vi "Agilent N6700 Series Configure Voltage.vi"() -> ()   [LabVIEW 2016]
doc: "Configures the power supply's output range on a channel, configures the DC voltage level, channel appears at the output connector and takes a measurement on the output signal and returns the measured value."
uses:
  <instrlib>/Agilent N6700 Series/Agilent N6700 Series.lvlib
panel:
  in  "Limit (1.0 A)":dbl=1.0 format="%^.3e"
  in  "Behavior (0: Regulatory Limit)":i32(ring) items=["Regulatory Limit", "Trip Limit"]
  out "Voltage Measurement":dbl format="%^.3e"
  in  "Voltage Level  (5.0 V)":dbl=5.0 format="%^.3e"
  in  "Voltage Range (10.0 V)":dbl=10.0 format="%^.3e"
  in  "Channel Name (1)":string="1"
  in  "VISA resource name":refnum<visa-resource-name>
  # "(c) 2004-2019  National Instruments.  ALL RIGHTS RESERVED."
  # "Agilent N6700 DC Power Supply"
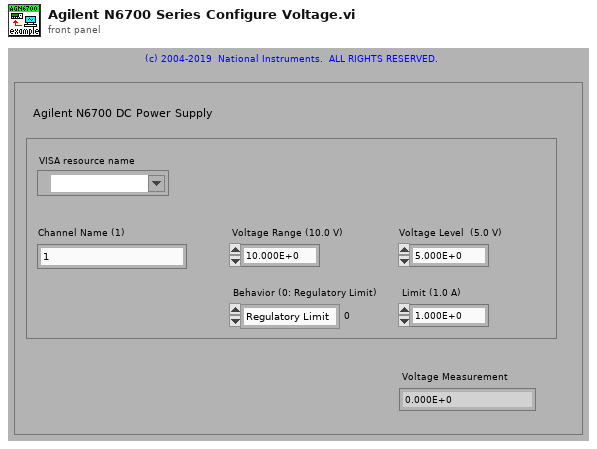
[diagram p1: front panel]
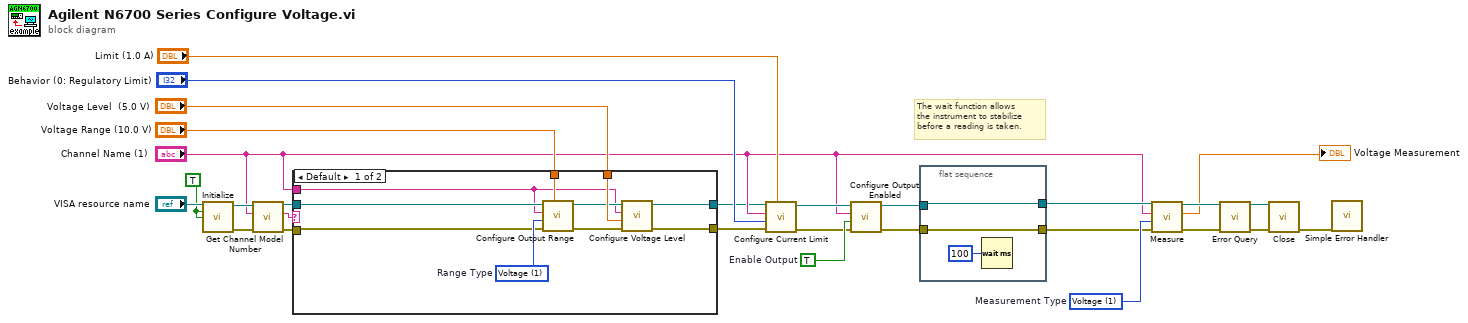
[diagram p0: block diagram]
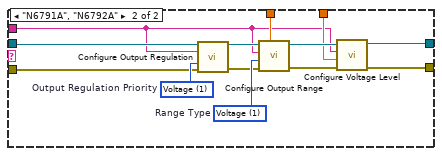
[diagram p2: hidden frame]
diagram:
  w18 = TRUE ("Reset? (T: Yes)")
  w19 = 1 items=["Voltage"=1, "Current"=0]  # Measurement Type
  w20 = TRUE  # Enable Output
  # "The wait function allows \nthe instrument to stabilize\nbefore a reading is taken."
  n1 = call <instrlib>:"Initialize.vi"("VISA resource name"="VISA resource name", "ID Query? (T: Yes)"=w18, "Reset? (T: Yes)"=w18) -> ("VISA resource name out"=w9:refnum<visa-resource-name>, "error out"=w8:errorcluster)  [unwired: 11 in]
  n2 = call <instrlib>:"Get Channel Model Number.vi"("error in (no error)"=w8, "Channel Name (1)"="Channel Name (1)", "VISA resource name"=w9) -> ("error out"=w6:errorcluster, "Model Number"=w5:string, "VISA resource name out"=w7:refnum<visa-resource-name>)  [unwired: 6 in]
  n3 = case shown="Default" w5 {
    tunnel: "Voltage Range (10.0 V)" -> [w35 w51]
    tunnel: "Channel Name (1)" -> [w29 w41]
    tunnel: w7 -> [w37 w46]
    tunnel: w6 -> [w36 w45]
    tunnel: "Voltage Level  (5.0 V)" -> [w33 w42]
    tunnel: [w31 w39] -> w2
    tunnel: [w30 w40] -> w1
    frame Default {
      w38 = 1 items=["Voltage"=1, "Current"=0]  # Range Type
      n4 = call <instrlib>:"Configure Output Range.vi"("Range (0.0)"=w35, "error in (no error)"=w36, "Range Type (1: Voltage)"=w38, "Channel Name (1)"=w29, "VISA resource name"=w37) -> ("error out"=w34:errorcluster, "VISA resource name out"=w32:refnum<visa-resource-name>)  [unwired: 5 in]
      n5 = call <instrlib>:"Configure Voltage Level.vi"("error in (no error)"=w34, "Level  (0.0 volts)"=w33, "Channel Name (1)"=w29, "VISA resource name"=w32) -> ("error out"=w31:errorcluster, "VISA resource name out"=w30:refnum<visa-resource-name>)  [unwired: 6 in]
    }
    frame "N6791A", "N6792A" {
      w47 = 1 items=["Voltage"=1, "Current"=0]  # Output Regulation Priority
      w50 = 1 items=["Voltage"=1, "Current"=0]  # Range Type
      n6 = call <instrlib>:"Configure Output Regulation.vi"("VISA resource name"=w46, "Channel Name (1)"=w41, "Output Regulation Priority (1: Voltage)"=w47, "error in (no error)"=w45) -> ("VISA resource name out"=w49:refnum<visa-resource-name>, "error out"=w48:errorcluster)  [unwired: 10 in]
      n7 = call <instrlib>:"Configure Output Range.vi"("Range (0.0)"=w51, "error in (no error)"=w48, "Range Type (1: Voltage)"=w50, "Channel Name (1)"=w41, "VISA resource name"=w49) -> ("error out"=w43:errorcluster, "VISA resource name out"=w44:refnum<visa-resource-name>)  [unwired: 5 in]
      n8 = call <instrlib>:"Configure Voltage Level.vi"("error in (no error)"=w43, "Level  (0.0 volts)"=w42, "Channel Name (1)"=w41, "VISA resource name"=w44) -> ("error out"=w39:errorcluster, "VISA resource name out"=w40:refnum<visa-resource-name>)  [unwired: 6 in]
    }
  }
  n9 = call <instrlib>:"Configure Current Limit.vi"("Limit (0.0 amps)"="Limit (1.0 A)", "error in (no error)"=w2, "Behavior (0: Regulatory Limit)"="Behavior (0: Regulatory Limit)", "Channel Name (1)"="Channel Name (1)", "VISA resource name"=w1) -> ("error out"=w17:errorcluster, "VISA resource name out"=w16:refnum<visa-resource-name>)  [unwired: 5 in]
  n10 = call <instrlib>:"Configure Output Enabled.vi"("error in (no error)"=w17, "Enable Output (False)"=w20, "Channel Name (1)"="Channel Name (1)", "VISA resource name"=w16) -> ("error out"=w10:errorcluster, "VISA resource name out"=w13:refnum<visa-resource-name>)  [unwired: 6 in]
  n11 = flat-sequence {
    tunnel: w13 -> [w54]
    tunnel: [w54] -> w12
    tunnel: [w52] -> w11
    tunnel: w10 -> [w52]
    frame #0 {
      n12 = Wait (ms)(milliseconds to wait=u32 100) -> ()  [unwired: 1 out]
    }
  }
  n13 = call <instrlib>:"Measure.vi"("error in (no error)"=w11, "Measurement Type (1: Voltage)"=w19, "Channel Name (1)"="Channel Name (1)", "VISA resource name"=w12) -> ("error out"=w27:errorcluster, "Measurement"=→"Voltage Measurement":dbl, "VISA resource name out"=w24:refnum<visa-resource-name>)  [unwired: 5 in]
  n14 = call <instrlib>:"Error Query.vi"("VISA resource name"=w24, "error in (no error)"=w27) -> ("VISA resource name out"=w25:refnum<visa-resource-name>, "error out"=w26:errorcluster)  [unwired: 10 in, 2 out]
  n15 = call <instrlib>:"Close.vi"("VISA resource name"=w25, "error in (no error)"=w26) -> ("error out"=w28:errorcluster)  [unwired: 13 in]
  n16 = call <vilib>:"Simple Error Handler.vi"("error in (no error)"=w28) -> ()  [unwired: 4 in, 5 out]
